vi "intitialize_map.vi"(11 "Map":enum16{"Grid"}(ring)) -> (1 "MapDistanceInfo":T1 {"Top Left Pixel UTM"."North" format="%#_10f"; "Top Left Pixel UTM"."East" format="%#_8f"; "Bottom Right Pixel UTM"."North" format="%#_10f"; "Bottom Right Pixel UTM"."East" format="%#_8f"}, 3 "Map Image Out":T3)   [LabVIEW 2013]
doc: "This vi initializes the map image for the simulator map view\n\nMaci Crowell\n4/5/2014"
uses:
  <vilib>/vision/Image Controls.llb/IMAQ Image.ctl
  cRIO_Code/Data/TypeDefs/UTM Location.ctl
  TypeDef/map_metadata.ctl
panel:
  out "Meters/pixel":dbl
  out "Bottom Right Pixel UTM":T2 {"North" format="%#_10f"; "East" format="%#_8f"}
  out "Top Left Pixel UTM":T2 {"North" format="%#_10f"; "East" format="%#_8f"}
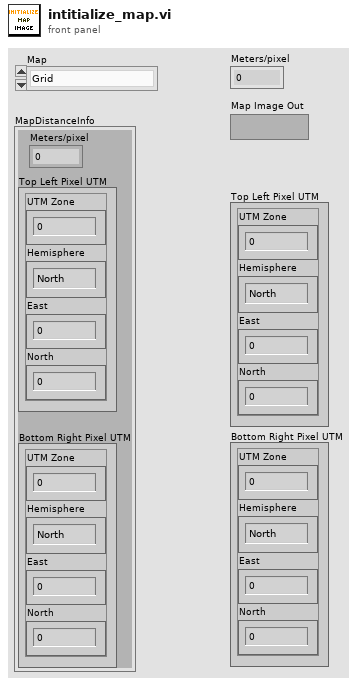
[diagram p1: front panel]
types:
  T1 = typedef "map_metadata.ctl" = cluster{"Meters/pixel":dbl, "Top Left Pixel UTM":T2, "Bottom Right Pixel UTM":T2}
  T2 = typedef "UTM Location.ctl" = cluster{"UTM Zone":dbl, "Hemisphere":enum16{"North", "South"}, "East":dbl, "North":dbl}
  T3 = typedef "IMAQ Image.ctl" = refnum<image>
  T4 = typedef "Image Type" = u32
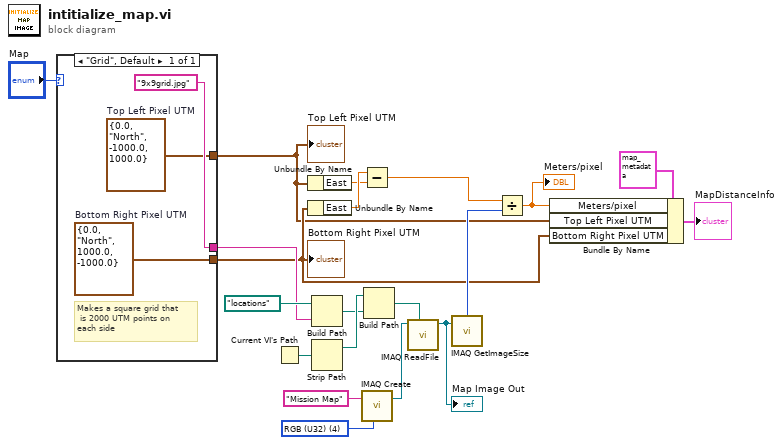
[diagram p0: block diagram]
diagram:
  w19 = T4 4 items=["Grayscale (U8)", "Grayscale (I16)", "Grayscale (SGL)", "Complex (CSG)", "RGB (U32)", "HSL (U32)", "RGB (U64)", "Grayscale (U16)"] ("Image Type")
  n1 = case shown="\"Grid\", Default" "Map" {
    tunnel: ["9x9grid.jpg"] -> w11
    tunnel: [w22] -> w4
    tunnel: [w21] -> w5
    frame "Grid", Default {
      w21 = T2 {"UTM Zone"=0.0, "Hemisphere"=enum."North", "East"=1000.0, "North"=-1000.0}  # Bottom Right Pixel UTM
      w22 = T2 {"UTM Zone"=0.0, "Hemisphere"=enum."North", "East"=-1000.0, "North"=1000.0}  # Top Left Pixel UTM
      # "Makes a square grid that\n is 2000 UTM points on \neach side"
    }
  }
  "Top Left Pixel UTM" <- w4
  "Bottom Right Pixel UTM" <- w5
  n2 = Current VI's Path() -> (path=w17:path)
  n3 = Unbundle By Name(w4) -> ("East"=w8:dbl)
  n4 = Unbundle By Name(w5) -> ("East"=w9:dbl)
  n5 = Build Path(base path=path "locations", name or relative path=w11) -> (appended path=w14:path)
  n6 = Strip Path(path=w17) -> (stripped path=w16:path)  [unwired: 1 out]
  n7 = Subtract(x=w9, y=w8) -> (x-y=w7:dbl)
  n8 = call "IMAQ Create"("Image Name"="Mission Map", "Image Type"=w19) -> ("New Image"=w18:T3)  [unwired: 2 in, 2 out]
  n9 = Build Path(base path=w16, name or relative path=w14) -> (appended path=w13:path)
  n10 = call "IMAQ ReadFile"("File Path"=w13, "Image"=w18) -> ("Image Out"=w10:T3)  [unwired: 3 in, 6 out]
  "Map Image Out" <- w10
  n11 = call "IMAQ GetImageSize"("Image"=w10) -> ("X Resolution"=w6:i32)  [unwired: 3 in, 2 out]
  n12 = Divide(x=w7, y=w6) -> (x/y=w3:dbl)
  "Meters/pixel" <- w3
  n13 = Bundle By Name(cluster=T1 {"Meters/pixel"=0.0, "Top Left Pixel UTM"={"UTM Zone"=0.0, "Hemisphere"=enum."North", "East"=0.0, "North"=0.0}, "Bottom Right Pixel UTM"={"UTM Zone"=0.0, "Hemisphere"=enum."North", "East"=0.0, "North"=0.0}} ("input cluster"), "Meters/pixel"=w3, "Top Left Pixel UTM"=w4, "Bottom Right Pixel UTM"=w5) -> (→"MapDistanceInfo":T1)
